vi "counterVarStep.vi"(0 "stepSize":u32, 1 "countMax":u32, 3 "doStep":bool=TRUE, 4 "reset":bool) -> (7 "index":u32, 8 "next":u32, 10 "maxReached":bool)   [LabVIEW 2016]
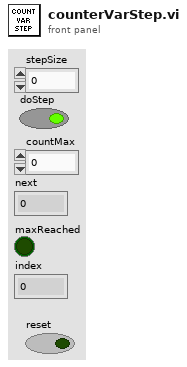
[diagram p1: front panel]
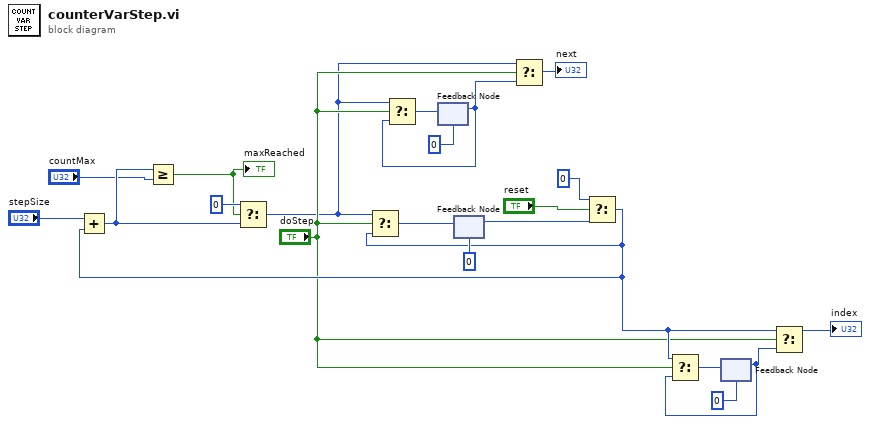
[diagram p0: block diagram]
diagram:
  n1 = feedback #1(u32 0 ("t")) -> (w1:u32)
  n2 = feedback #2(u32 0 ("t")) -> (w14:u32)
  n3 = Select(t=u32 0, s="reset", f=w14) -> (s? t:f=w8:u32)
  n4 = Add(x="stepSize", y=w8) -> (x+y=w19:u32)
  n5 = Greater Or Equal?(x=w19, y="countMax") -> (x >= y?=w17:bool)
  "maxReached" <- w17
  n6 = Select(t=u32 0, s=w17, f=w19) -> (s? t:f=w2:u32)
  n7 = Select(t=w2, s="doStep", f=w8) -> (s? t:f=w13:u32)
  n8 = Select(t=w2, s="doStep", f=w1) -> (s? t:f=w4:u32)
  n9 = feedback-in #1(w4) -> ()
  n10 = feedback-in #2(w13) -> ()
  n11 = Select(t=w2, s="doStep", f=w1) -> (s? t:f=→"next":u32)
  n12 = feedback #3(u32 0 ("t")) -> (w7:u32)
  n13 = Select(t=w8, s="doStep", f=w7) -> (s? t:f=w9:u32)
  n14 = feedback-in #3(w9) -> ()
  n15 = Select(t=w8, s="doStep", f=w7) -> (s? t:f=→"index":u32)
